vi "q1 random integers.vi"() -> ()   [LabVIEW 2025]
panel:
  out "random":dbl[](array[numeric])
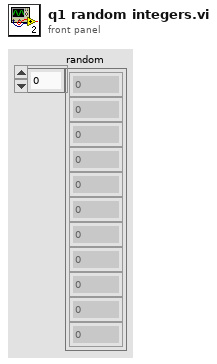
[diagram p1: front panel]
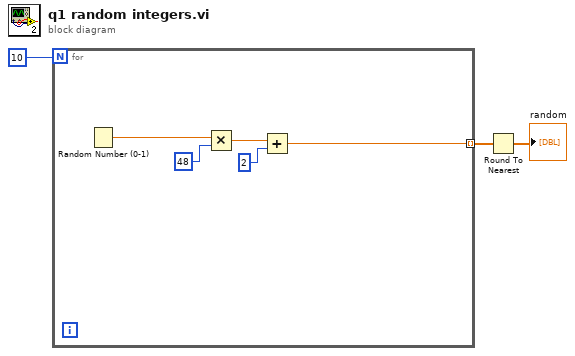
[diagram p0: block diagram]
diagram:
  n1 = for {
    N: 10 -> [_]
    tunnel: [w4] -> w2 mode=indexing
    n2 = Random Number (0-1)() -> (number: 0 to 1=w8:dbl)
    n3 = Multiply(x=w8, y=48) -> (x*y=w6:dbl)
    n4 = Add(x=w6, y=2) -> (x+y=w4:dbl)
  }
  n5 = Round To Nearest(number=w2) -> (nearest integer value=→"random":dbl[])
